vi "perc tri.vi"(0 "C":dbl[][](array[numeric]), 1 "trigger":i32, 2 "B":dbl[][](array[numeric]), 3 "A":dbl[][](array[numeric]), 4 "%":dbl) -> (5 "Array":dbl[][](array[numeric]))   [LabVIEW 2018]
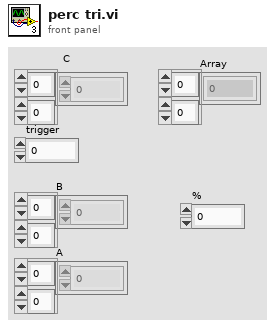
[diagram p1: front panel]
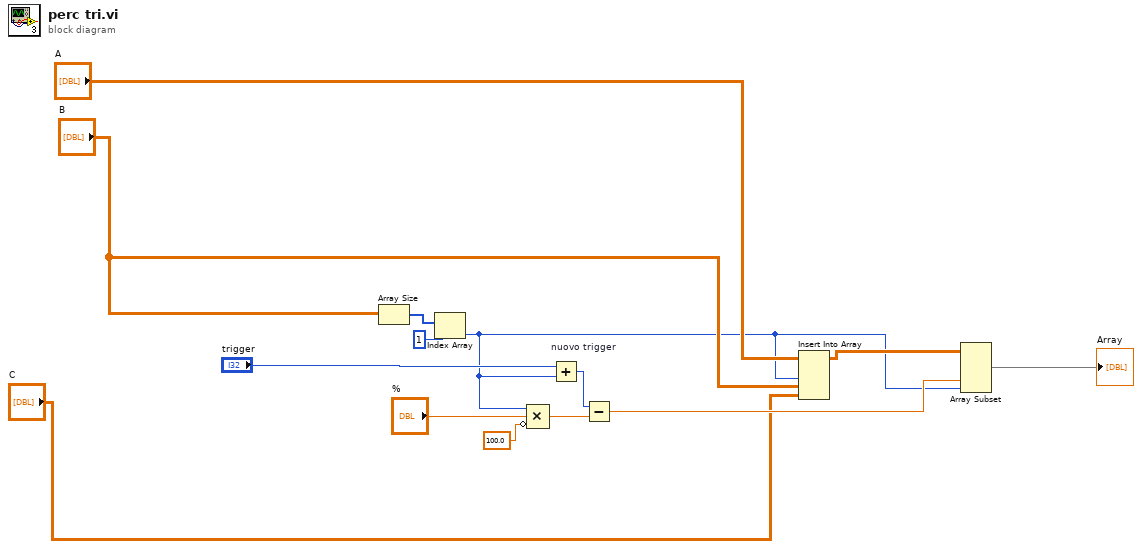
[diagram p0: block diagram]
diagram:
  n1 = Array Size(array="B") -> (size(s)=w9:i32[])
  n2 = Index Array(array=w9, index=1) -> (element=w1:i32)
  n3 = Compound Arithmetic op=MULTIPLY(w1, "%", invert 100.0 ("value")) -> (w10:dbl)
  n4 = Add "nuovo trigger"(x="trigger", y=w1) -> (x+y=w14:i32)
  n5 = Subtract(x=w14, y=w10) -> (x-y=w7:dbl)
  n6 = Insert Into Array(array="A", index (col)=w1, new element #1="B", new element #2="C") -> (w5:dbl[][])  [unwired: 1 in]
  n7 = Array Subset(array=w5, index (col)=w7, length (col)=w1) -> (→"Array":dbl[][])  [unwired: 2 in]
